vi "GetType.vi"(8 "error in (no error)":errorcluster, 11 "Configure Multi-Point [MP] Msg":refnum<class "Configure Multi-Point [MP] Msg.lvclass">) -> (0 "error out":errorcluster, 2 "Data Sample":variant, 3 "Configure Multi-Point [MP] Msg":refnum<class "Configure Multi-Point [MP] Msg.lvclass">)   [LabVIEW 2016, in "CS++DMM.lvlib" / "Configure Multi-Point [MP] Msg.lvclass"]
uses:
  Configure Multi-Point [MP] Msg.lvclass
  Configure Multi-Point [MP] Msg.lvclass/Configure Multi-Point [MP] Msg.ctl
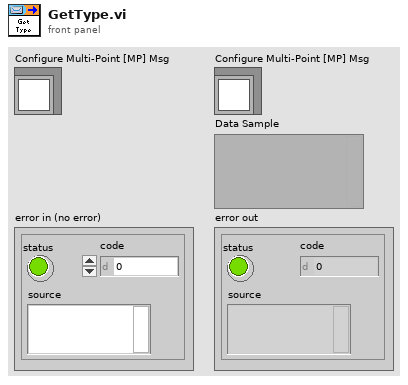
[diagram p1: front panel]
types:
  T1 = cluster{"trigger count (1)":i32, "sample count (1)":i32, "sample trigger (Immediate)":i32, "sample interval (0.0 s)":dbl}
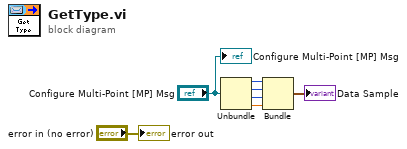
[diagram p0: block diagram]
diagram:
  n1 = Unbundle("Configure Multi-Point [MP] Msg") -> (w4:i32, w3:i32, w2:i32, w1:dbl)
  n2 = Bundle("trigger count (1)"=w4, "sample count (1)"=w3, "sample trigger (Immediate)"=w2, "sample interval (0.0 s)"=w1) -> (→"Data Sample":T1)  [unwired: 1 in]
  "error out" <- "error in (no error)"
  "Configure Multi-Point [MP] Msg" <- "Configure Multi-Point [MP] Msg"
